vi "Acq&Buf-module5761.vi"(0 "DMATtoHOSTBlockNWords":u16, 1 "IntermediateFIFO":refnum<k21>="FIFO0", 2 "BUFFERS Info":T2={"CH0BUFFER"="CH0BUFFER", "CH1BUFFER"="CH1BUFFER", "CH2BUFFER"="CH2BUFFER", "CH3BUFFER"="CH3BUFFER", "CH0DMANumber "=0, "CH1DMANumber"=0, "CH2DMANumber"=0, "CH3DMANumber"=0}, 3 "DMA number":i32, 5 "SamplingRateN(DecimationFactor)":u16, 7 "NumberOfBuffers":T1, 9 "GroupEnableN":bool, 11 "DebugActivation":bool, 12 "Selected Channels":T4[](array[typedef])=[enum."Empty", enum."Empty", enum."Empty", enum."Empty"], 13 "NumChannels":T3) -> ()   [LabVIEW 2013, in "IRIO.lvlib"]
uses:
  IRIO.lvlib
  common/GlobalReg.vi
  <vilib>/eio/EIONode/EIONode.xnode
  <vilib>/rvi/eio/common/nirviEmuTemplateMethod_errors.vi
  <vilib>/rvi/DataTransferAndStorage/Container/XNode/niFpgaContainer.xnode
  <vilib>/rvi/FIFO/Fifo_Resource/niFpgaFifoEmulationRefIn.vi
  <vilib>/rvi/LocalResourceManager/LocalResourceManager.xnode
  <vilib>/rvi/DataTransferAndStorage/Container/Common/niFpgaContainerGetUniqueNameForEmu.vi
  <vilib>/rvi/DataTransferAndStorage/Container/Common/niFpgaContainerSetEmuInfo.vi
  <vilib>/rvi/eio/common/nirviEmuReportErrorAndStop.vi
  <vilib>/rvi/DataTransferAndStorage/Register/Emulation/niFpgaRegisterEmulationRefIn.vi
  ctl/SelectedChannels.ctl
  ctl/DMAConfigParams.ctl
  ctl/NumberOfBuffers.ctl
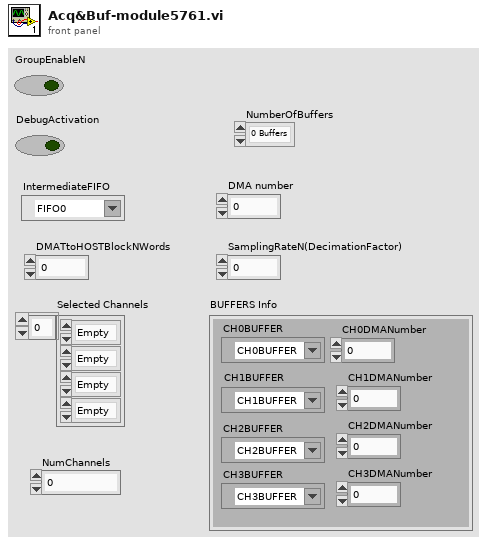
[diagram p1: front panel]
types:
  T1 = typedef "IRIO.lvlib/NumberOfBuffers.ctl" = enum16{"0 Buffers", "1 Buffers", "2 Buffers", "3 Buffers", "4 Buffers", "5 Buffers", "6 Buffers", "7 Buffers", "8 Buffers", "9 Buffers", "10 Buffers", "11 Buffers", "12 Buffers"}
  T2 = cluster{"CH0BUFFER":refnum<k21>, "CH1BUFFER":refnum<k21>, "CH2BUFFER":refnum<k21>, "CH3BUFFER":refnum<k21>, "CH0DMANumber ":i32, "CH1DMANumber":i32, "CH2DMANumber":i32, "CH3DMANumber":i32}
  T3 = typedef "IRIO.lvlib/DMAConfigParams.ctl" = u16
  T4 = typedef "IRIO.lvlib/SelectedChannels.ctl" = enum16{"Empty", "AI0", "AI1", "AI2", "AI3", "SignalGenerator0", "SignalGenerator1", "DDCA_PORT0", "DDCA_PORT1", "DDCA_PORT2", "DDCB_PORT0", "DDCB_PORT1", "DDCB_PORT2"}
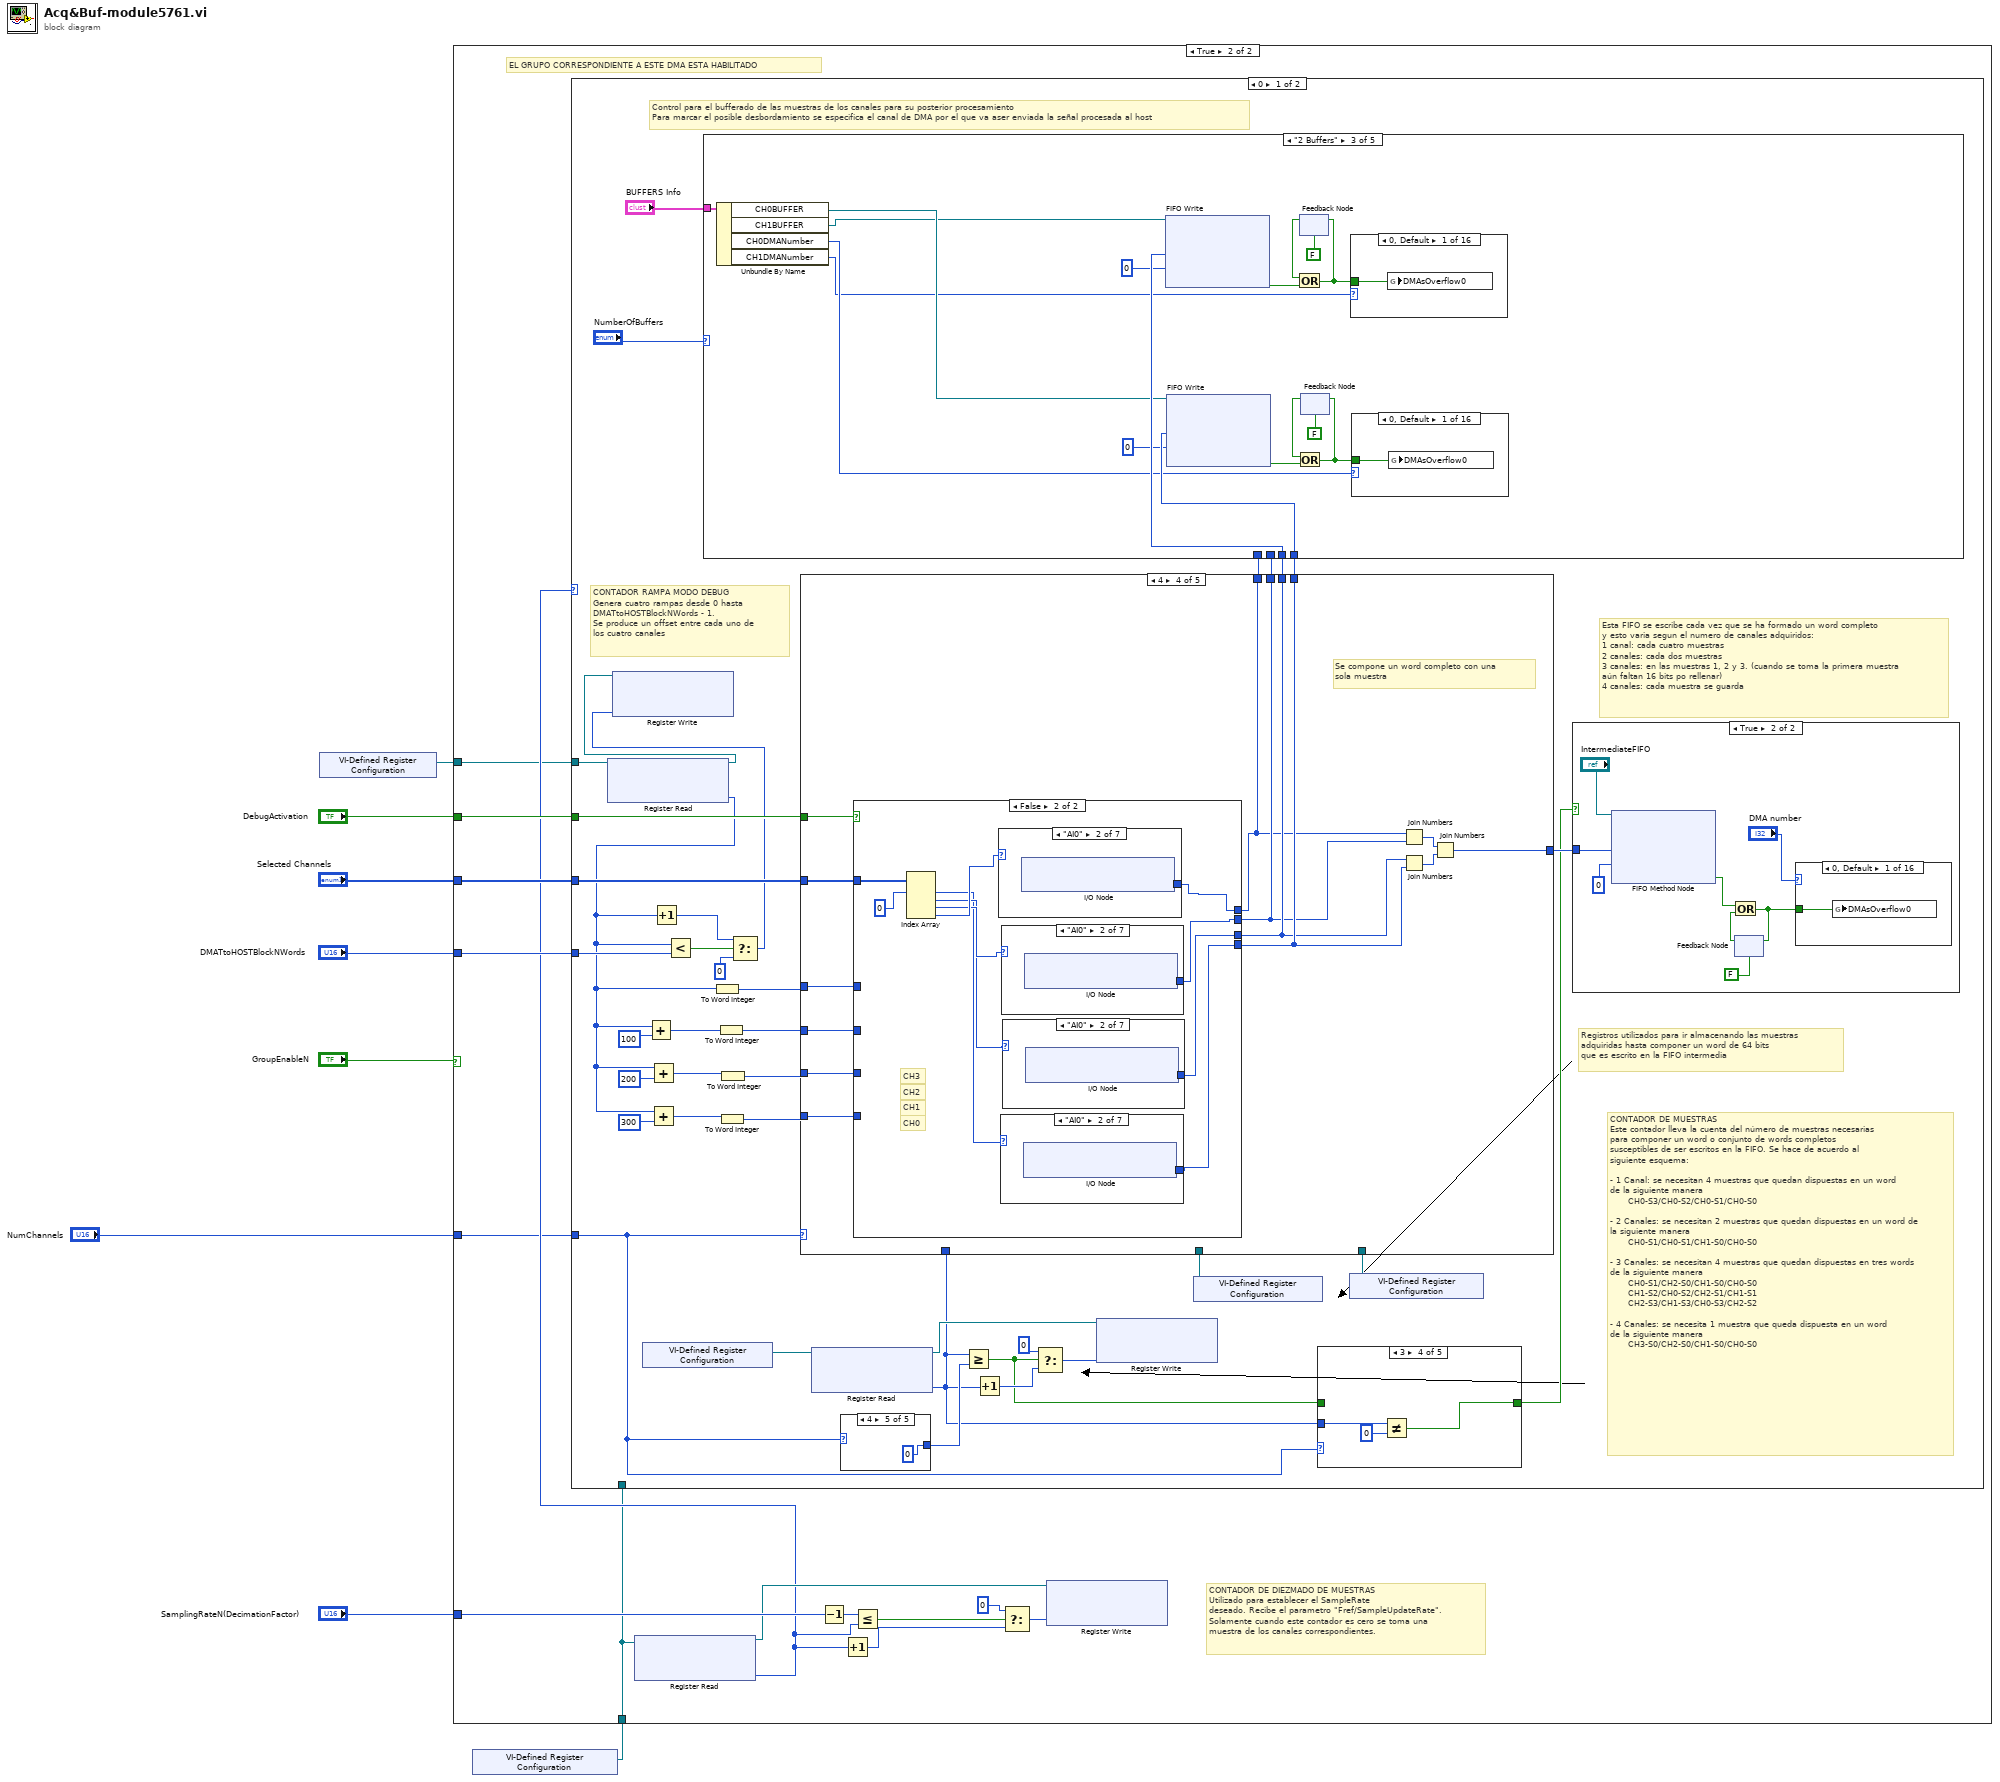
[diagram p0: block diagram]
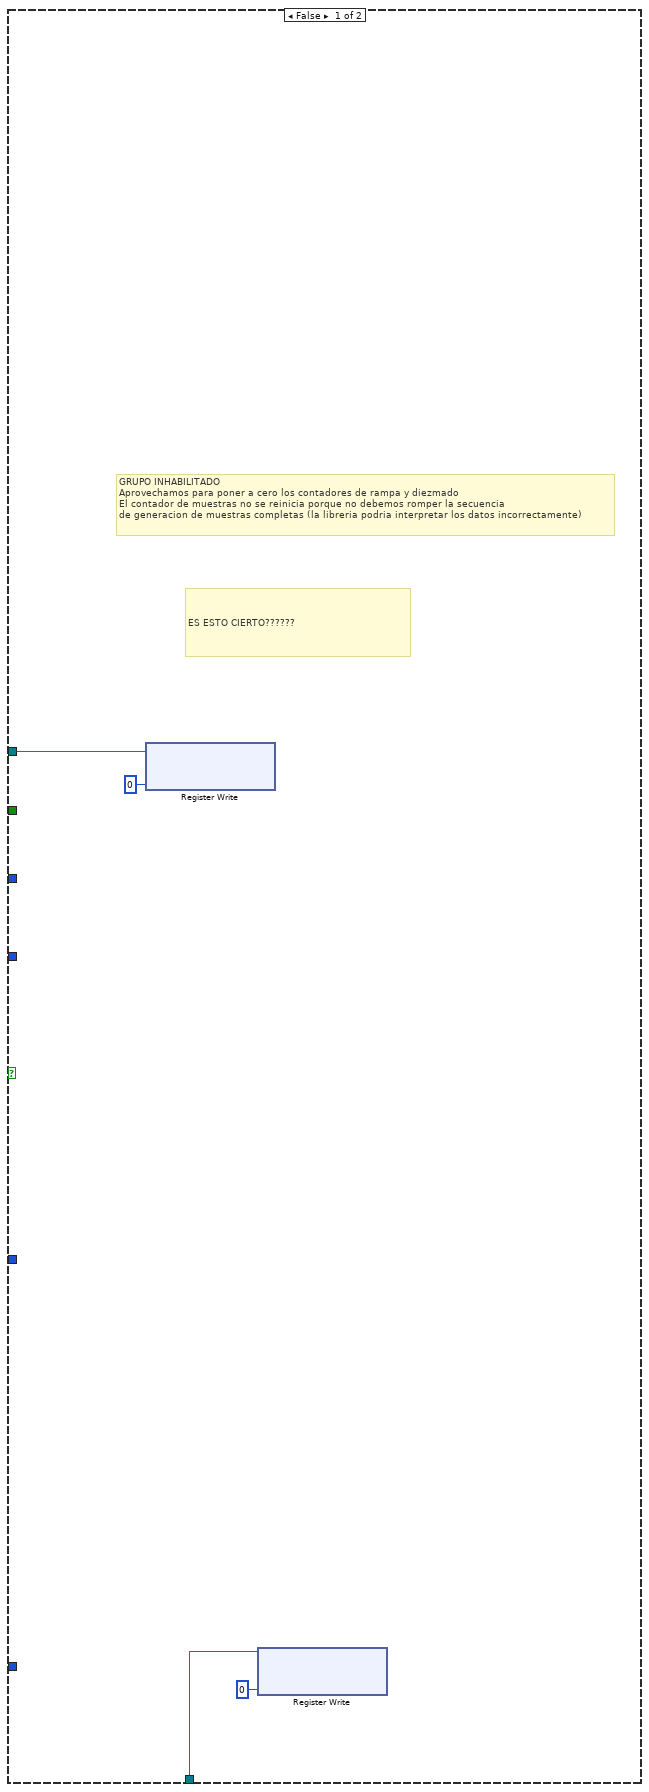
[diagram p2: hidden frame]
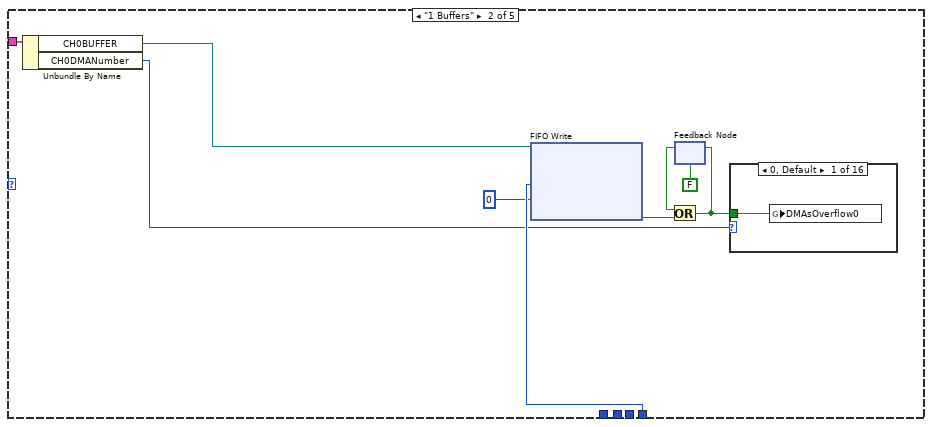
[diagram p4: hidden frame]
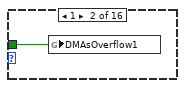
[diagram p5: hidden frame]
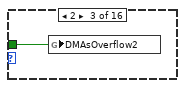
[diagram p6: hidden frame]
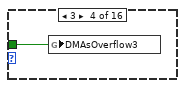
[diagram p7: hidden frame]
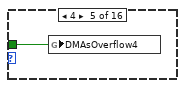
[diagram p8: hidden frame]
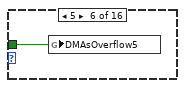
[diagram p9: hidden frame]
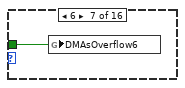
[diagram p10: hidden frame]
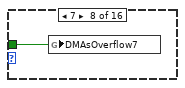
[diagram p11: hidden frame]
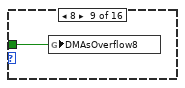
[diagram p12: hidden frame]
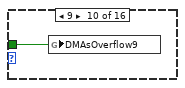
[diagram p13: hidden frame]
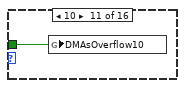
[diagram p14: hidden frame]
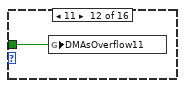
[diagram p15: hidden frame]
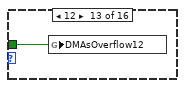
[diagram p16: hidden frame]
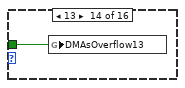
[diagram p17: hidden frame]
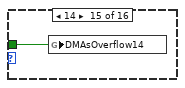
[diagram p18: hidden frame]
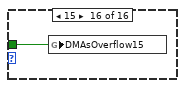
[diagram p19: hidden frame]
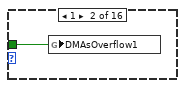
[diagram p20: hidden frame]
diagram:
  n1 = xnode ("VI-Defined Register Configuration")() -> ("Register Out"=w2:refnum<k21>)
  n2 = xnode ("VI-Defined Register Configuration")() -> ("Register Out"=w3:refnum<k21>)
  n3 = case shown="True" "GroupEnableN" {
    tunnel: "DebugActivation" -> [_ w26]
    tunnel: "DMATtoHOSTBlockNWords" -> [_ w25]
    tunnel: "NumChannels" -> [_ w13]
    tunnel: "Selected Channels" -> [_ w24]
    tunnel: "SamplingRateN(DecimationFactor)" -> [_ w19]
    tunnel: w3 -> [w12 w15]
    tunnel: w2 -> [w10 w14]
    frame False {
      # "ES ESTO CIERTO??????"
      # "GRUPO INHABILITADO\nAprovechamos para poner a cero los contadores de rampa y diezmado\nEl contador de muestras no se reinicia porque no debemos romper la secuencia\nde generacion de muestras completas (la libreria podria interpretar los datos incorrectamente)"
      n4 = xnode ("Register Write")("Data"=u16 0, "Register In"=w10) -> ()  [unwired: 1 out]
      n5 = xnode ("Register Write")("Data"=u16 0, "Register In"=w12) -> ()  [unwired: 1 out]
    }
    frame True {
      # "EL GRUPO CORRESPONDIENTE A ESTE DMA ESTA HABILITADO"
      # "CONTADOR DE DIEZMADO DE MUESTRAS\nUtilizado para establecer el SampleRate \ndeseado. Recibe el parametro \"Fref/SampleUpdateRate\".\nSolamente cuando este contador es cero se toma una\nmuestra de los canales correspondientes."
      n6 = xnode ("Register Read")("Register In"=w15) -> ("Register Out"=w18:refnum<k21>, "Data"=w16:u16)
      n7 = case shown="0" w16 {
        tunnel: w26 -> [w65 _]
        tunnel: w25 -> [w60 _]
        tunnel: w13 -> [w52 _]
        tunnel: w24 -> [w63 _]
        tunnel: w15 -> [_ _]
        tunnel: w14 -> [w45 _]
        frame 0 {
          # "Control para el bufferado de las muestras de los canales para su posterior procesamiento\nPara marcar el posible desbordamiento se especifica el canal de DMA por el que va aser enviada la señal procesada al host"
          # "Esta FIFO se escribe cada vez que se ha formado un word completo\ny esto varia segun el numero de canales adquiridos: \n1 canal: cada cuatro muestras\n2 canales: cada dos muestras\n3 canales: en las muestras 1, 2 y 3. (cuando se toma la primera muestra\naún faltan 16 bits po rellenar)\n4 canales: cada muestra se guarda"
          # "CONTADOR DE MUESTRAS\nEste contador lleva la cuenta del número de muestras necesarias\npara componer un word o conjunto de words completos\nsusceptibles de ser escritos en la FIFO. Se hace de acuerdo al\nsiguiente esquema:\n\n- 1 Canal: se necesitan 4 muestras que quedan dispuestas en un word \nde la siguiente manera\n      CH0-S3/CH0-S2/CH0-S1/CH0-S0\n\n- 2 Canales: se necesitan 2 muestras que quedan dispuestas en un word de la siguiente manera\n      CH0-S1/CH0-S1/CH1-S0/CH0-S0\n\n- 3 Canales: se necesitan 4 muestras que quedan dispuestas en tres words de la siguiente manera\n      CH0-S1/CH2-S0/CH1-S0/CH0-S0\n      CH1-S2/CH0-S2/CH2-S1/CH1-S1\n      CH2-S3/CH1-S3/CH0-S3/CH2-S2\n\n- 4 Canales: se necesita 1 muestra que queda dispuesta en un word \nde la siguiente manera\n      CH3-S0/CH2-S0/CH1-S0/CH0-S0"
          # "Registros utilizados para ir almacenando las muestras\nadquiridas hasta componer un word de 64 bits\nque es escrito en la FIFO intermedia"
          # "CONTADOR RAMPA MODO DEBUG\nGenera cuatro rampas desde 0 hasta \nDMATtoHOSTBlockNWords - 1.\nSe produce un offset entre cada uno de \nlos cuatro canales"
          n8 = xnode ("Register Read")("Register In"=w45) -> ("Data"=w33:u16, "Register Out"=w44:refnum<k21>)
          n9 = xnode ("VI-Defined Register Configuration")() -> ("Register Out"=w48:refnum<k21>)
          n10 = Add(x=w33, y=u16 100) -> (x+y=w40:u16)
          n11 = Add(x=w33, y=u16 200) -> (x+y=w38:u16)
          n12 = Add(x=w33, y=u16 300) -> (x+y=w36:u16)
          n13 = Increment(x=w33) -> (x+1=w62:u16)
          n14 = Less?(x=w33, y=w60) -> (x < y?=w61:bool)
          n15 = To Word Integer(number=w33) -> (16bit integer=w41:i16)
          n16 = To Word Integer(number=w40) -> (16bit integer=w39:i16)
          n17 = To Word Integer(number=w36) -> (16bit integer=w35:i16)
          n18 = To Word Integer(number=w38) -> (16bit integer=w37:i16)
          n19 = Select(t=w62, s=w61, f=u16 0) -> (s? t:f=w43:u16)
          n20 = xnode ("Register Write")("Data"=w43, "Register In"=w44) -> ()  [unwired: 1 out]
          n21 = xnode ("Register Read")("Register In"=w48) -> ("Register Out"=w53:refnum<k21>, "Data"=w49:u8)
          n22 = case shown="4" w52 {
            tunnel: [u8 0 u8 3 u8 1 u8 3 u8 0] -> w54
            frame 0, Default {
            }
            frame 1 {
            }
            frame 2 {
            }
            frame 3 {
            }
            frame 4 {
            }
          }
          n23 = Greater Or Equal?(x=w49, y=w54) -> (x >= y?=w51:bool)
          n24 = Increment(x=w49) -> (x+1=w57:u8)
          n25 = Select(t=u8 0 ("f"), s=w51, f=w57) -> (s? t:f=w55:u8)
          n26 = xnode ("Register Write")("Data"=w55, "Register In"=w53) -> ()  [unwired: 1 out]
          n27 = xnode ("VI-Defined Register Configuration")() -> ("Register Out"=w47:refnum<k21>)
          n28 = case shown="3" w52 {
            tunnel: w51 -> [_ w311 w312 _ w316]
            tunnel: [FALSE w311 w312 w313 w316] -> w50
            tunnel: w49 -> [_ _ _ w315 _]
            frame 0, Default {
            }
            frame 1 {
            }
            frame 2 {
            }
            frame 3 {
              n29 = Not Equal?(x=w315, y=u8 0) -> (x != y?=w313:bool)
            }
            frame 4 {
            }
          }
          n30 = xnode ("VI-Defined Register Configuration")() -> ("Register Out"=w46:refnum<k21>)
          n31 = case shown="4" w52 {
            tunnel: w65 -> [w354 w407 w459 w559 _]
            tunnel: w41 -> [w351 w404 w456 w558 _]
            tunnel: [w352 w405 w457 w554 u64 0] -> w64
            tunnel: w63 -> [w353 w406 w458 w557 _]
            tunnel: w39 -> [w350 w403 w455 w553 _]
            tunnel: w37 -> [_ _ w454 w552 _]
            tunnel: w35 -> [_ _ _ w551 _]
            tunnel: w49 -> [w349 w402 w453 _ _]
            tunnel: w47 -> [_ _ w452 _ _]
            tunnel: w46 -> [w348 w401 w451 _ _]
            tunnel: [w347 w400 w450 w550 w610] -> w32
            tunnel: [w346 w399 w449 w549 w610] -> w31
            tunnel: [w346 w398 w448 w548 w610] -> w30
            tunnel: [w346 w398 i16 0 ("IO Module\\AI 0") w547 w610] -> w29
            frame 1 {
              w346 = i16 0 ("IO Module\\AI 0")
              # "Cada muestra se va guardando en un registro intermedio\nhasta componer los 64 bits"
              n32 = case shown="False" w354 {
                tunnel: w353 -> [w357 _]
                tunnel: [w355 w368] -> w347
                tunnel: w351 -> [_ w368]
                tunnel: w350 -> [_ _]
                frame False {
                  n33 = Index Array(array=w357, index=0) -> (element=w356:T4)
                  n34 = case shown="\"AI0\"" w356 {
                    tunnel: [i16 0 ("IO Module\\AI 0") w360 w361 w362 w363 w365 w367] -> w355
                    frame "Empty", Default {
                    }
                    frame "AI0" {
                      n35 = xnode "I/O Node"() -> ("IO Module\\AI 0 Data N"=w360)  [unwired: 1 in, 1 out]
                    }
                    frame "AI1" {
                      n36 = xnode "I/O Node"() -> ("IO Module\\AI 1 Data N"=w361)  [unwired: 1 in, 1 out]
                    }
                    frame "AI2" {
                      n37 = xnode "I/O Node"() -> ("IO Module\\AI 2 Data N"=w362)  [unwired: 1 in, 1 out]
                    }
                    frame "AI3" {
                      n38 = xnode "I/O Node"() -> ("IO Module\\AI 3 Data N"=w363)  [unwired: 1 in, 1 out]
                    }
                    frame "SignalGenerator0" {
                      n39 = global read "GlobalReg.vi" "SimulatedAO0"() -> (w364:i32)
                      n40 = To Word Integer(number=w364) -> (16bit integer=w365:i16)
                    }
                    frame "SignalGenerator1" {
                      n41 = global read "GlobalReg.vi" "SimulatedAO1"() -> (w366:i32)
                      n42 = To Word Integer(number=w366) -> (16bit integer=w367:i16)
                    }
                  }
                }
                frame True {
                }
              }
              n43 = case shown="0, Default" w349 {
                tunnel: w347 -> [w371 w380 w387 w397]
                tunnel: [w370 w378 w385 w394] -> w352
                tunnel: w348 -> [w369 w377 w384 w392]
                frame 1 {
                  n44 = xnode ("Register Read")("Register In"=w369) -> ("Data"=w376:u64)  [unwired: 1 out]
                  n45 = Split Number(x=w376) -> (lo(x)=w375:u32)  [unwired: 1 out]
                  n46 = Split Number(x=w375) -> (lo(x)=w372:u16)  [unwired: 1 out]
                  n47 = Join Numbers(hi=w371, lo=w372) -> ((hi.lo)=w374:u32)
                  n48 = Join Numbers(hi=u32 0, lo=w374) -> ((hi.lo)=w370:u64)
                  n49 = xnode ("Register Write")("Data"=w370, "Register In"=w369) -> ()  [unwired: 1 out]
                }
                frame 2 {
                  n50 = xnode ("Register Read")("Register In"=w377) -> ("Data"=w383:u64)  [unwired: 1 out]
                  n51 = Split Number(x=w383) -> (lo(x)=w382:u32)  [unwired: 1 out]
                  n52 = Join Numbers(hi=u16 0, lo=w380) -> ((hi.lo)=w381:u32)
                  n53 = Join Numbers(hi=w381, lo=w382) -> ((hi.lo)=w378:u64)
                  n54 = xnode ("Register Write")("Data"=w378, "Register In"=w377) -> ()  [unwired: 1 out]
                }
                frame 3 {
                  n55 = xnode ("Register Read")("Register In"=w384) -> ("Data"=w391:u64)  [unwired: 1 out]
                  n56 = Split Number(x=w391) -> (hi(x)=w388:u32, lo(x)=w390:u32)
                  n57 = Split Number(x=w388) -> (lo(x)=w386:u16)  [unwired: 1 out]
                  n58 = Join Numbers(hi=w387, lo=w386) -> ((hi.lo)=w389:u32)
                  n59 = Join Numbers(hi=w389, lo=w390) -> ((hi.lo)=w385:u64)
                }
                frame 0, Default {
                  n60 = Join Numbers(hi=u16 0, lo=w397) -> ((hi.lo)=w396:u32)
                  n61 = Join Numbers(hi=u32 0, lo=w396) -> ((hi.lo)=w394:u64)
                  n62 = xnode ("Register Write")("Data"=w394, "Register In"=w392) -> ()  [unwired: 1 out]
                }
              }
            }
            frame 2 {
              w398 = i16 0 ("IO Module\\AI 0")
              # "Cada muestra de dos canales se van guardando en un registro\nintermedio hasta componer los 64 bits"
              n63 = case shown="False" w407 {
                tunnel: w406 -> [w412 _]
                tunnel: [w409 w433] -> w400
                tunnel: [w408 w432] -> w399
                tunnel: w404 -> [_ w433]
                tunnel: w403 -> [_ w432]
                frame False {
                  n64 = Index Array(array=w412, index #1=0 ("index")) -> (element #1=w411:T4, element #2=w410:T4)  [unwired: 1 in]
                  n65 = case shown="\"AI0\"" w411 {
                    tunnel: [i16 0 ("IO Module\\AI 0") w424 w425 w426 w427 w429 w431] -> w409
                    frame "Empty", Default {
                    }
                    frame "AI0" {
                      n66 = xnode "I/O Node"() -> ("IO Module\\AI 0 Data N"=w424)  [unwired: 1 in, 1 out]
                    }
                    frame "AI1" {
                      n67 = xnode "I/O Node"() -> ("IO Module\\AI 1 Data N"=w425)  [unwired: 1 in, 1 out]
                    }
                    frame "AI2" {
                      n68 = xnode "I/O Node"() -> ("IO Module\\AI 2 Data N"=w426)  [unwired: 1 in, 1 out]
                    }
                    frame "AI3" {
                      n69 = xnode "I/O Node"() -> ("IO Module\\AI 3 Data N"=w427)  [unwired: 1 in, 1 out]
                    }
                    frame "SignalGenerator0" {
                      n70 = global read "GlobalReg.vi" "SimulatedAO0"() -> (w428:i32)
                      n71 = To Word Integer(number=w428) -> (16bit integer=w429:i16)
                    }
                    frame "SignalGenerator1" {
                      n72 = global read "GlobalReg.vi" "SimulatedAO1"() -> (w430:i32)
                      n73 = To Word Integer(number=w430) -> (16bit integer=w431:i16)
                    }
                  }
                  n74 = case shown="\"AI0\"" w410 {
                    tunnel: [i16 0 ("IO Module\\AI 0") w415 w416 w417 w418 w420 w422] -> w408
                    frame "Empty", Default {
                    }
                    frame "AI0" {
                      n75 = xnode "I/O Node"() -> ("IO Module\\AI 0 Data N"=w415)  [unwired: 1 in, 1 out]
                    }
                    frame "AI1" {
                      n76 = xnode "I/O Node"() -> ("IO Module\\AI 1 Data N"=w416)  [unwired: 1 in, 1 out]
                    }
                    frame "AI2" {
                      n77 = xnode "I/O Node"() -> ("IO Module\\AI 2 Data N"=w417)  [unwired: 1 in, 1 out]
                    }
                    frame "AI3" {
                      n78 = xnode "I/O Node"() -> ("IO Module\\AI 3 Data N"=w418)  [unwired: 1 in, 1 out]
                    }
                    frame "SignalGenerator0" {
                      n79 = global read "GlobalReg.vi" "SimulatedAO0"() -> (w419:i32)
                      n80 = To Word Integer(number=w419) -> (16bit integer=w420:i16)
                    }
                    frame "SignalGenerator1" {
                      n81 = global read "GlobalReg.vi" "SimulatedAO1"() -> (w421:i32)
                      n82 = To Word Integer(number=w421) -> (16bit integer=w422:i16)
                    }
                  }
                }
                frame True {
                }
              }
              n83 = case shown="0, Default" w402 {
                tunnel: w400 -> [w440 w446]
                tunnel: w399 -> [w439 w445]
                tunnel: [w437 w442] -> w405
                tunnel: w401 -> [w434 w441]
                frame 1 {
                  n84 = xnode ("Register Read")("Register In"=w434) -> ("Data"=w438:u64)  [unwired: 1 out]
                  n85 = Join Numbers(hi=w439, lo=w440) -> ((hi.lo)=w435:u32)
                  n86 = Split Number(x=w438) -> (lo(x)=w436:u32)  [unwired: 1 out]
                  n87 = Join Numbers(hi=w435, lo=w436) -> ((hi.lo)=w437:u64)
                }
                frame 0, Default {
                  n88 = Join Numbers(hi=w445, lo=w446) -> ((hi.lo)=w444:u32)
                  n89 = Join Numbers(hi=u32 0, lo=w444) -> ((hi.lo)=w442:u64)
                  n90 = xnode ("Register Write")("Data"=w442, "Register In"=w441) -> ()  [unwired: 1 out]
                }
              }
            }
            frame 3 {
              # "Se necesitan dos registros porque las muestras de los tres canales\nen ocasiones quedan distribuidas entre dos word consecutivas. Cada\nuno de los tres words que se van generando se van escribiendo\nen la FIFO en el ciclo en el que se termina de componer"
              n91 = case shown="False" w459 {
                tunnel: w458 -> [w466 _]
                tunnel: [w465 w497] -> w450
                tunnel: [w464 w496] -> w449
                tunnel: w456 -> [_ w497]
                tunnel: w455 -> [_ w496]
                tunnel: [w463 w495] -> w448
                tunnel: w454 -> [_ w495]
                frame False {
                  n92 = Index Array(array=w466, index #1=0 ("index")) -> (element #1=w462:T4, element #2=w460:T4, element #3=w461:T4)  [unwired: 2 in]
                  n93 = case shown="\"AI0\"" w461 {
                    tunnel: [i16 0 ("IO Module\\AI 0") w469 w470 w471 w472 w474 w476] -> w463
                    frame "Empty", Default {
                    }
                    frame "AI0" {
                      n94 = xnode "I/O Node"() -> ("IO Module\\AI 0 Data N"=w469)  [unwired: 1 in, 1 out]
                    }
                    frame "AI1" {
                      n95 = xnode "I/O Node"() -> ("IO Module\\AI 1 Data N"=w470)  [unwired: 1 in, 1 out]
                    }
                    frame "AI2" {
                      n96 = xnode "I/O Node"() -> ("IO Module\\AI 2 Data N"=w471)  [unwired: 1 in, 1 out]
                    }
                    frame "AI3" {
                      n97 = xnode "I/O Node"() -> ("IO Module\\AI 3 Data N"=w472)  [unwired: 1 in, 1 out]
                    }
                    frame "SignalGenerator0" {
                      n98 = global read "GlobalReg.vi" "SimulatedAO0"() -> (w473:i32)
                      n99 = To Word Integer(number=w473) -> (16bit integer=w474:i16)
                    }
                    frame "SignalGenerator1" {
                      n100 = global read "GlobalReg.vi" "SimulatedAO1"() -> (w475:i32)
                      n101 = To Word Integer(number=w475) -> (16bit integer=w476:i16)
                    }
                  }
                  n102 = case shown="\"AI0\"" w462 {
                    tunnel: [i16 0 ("IO Module\\AI 0") w487 w488 w489 w490 w492 w494] -> w465
                    frame "Empty", Default {
                    }
                    frame "AI0" {
                      n103 = xnode "I/O Node"() -> ("IO Module\\AI 0 Data N"=w487)  [unwired: 1 in, 1 out]
                    }
                    frame "AI1" {
                      n104 = xnode "I/O Node"() -> ("IO Module\\AI 1 Data N"=w488)  [unwired: 1 in, 1 out]
                    }
                    frame "AI2" {
                      n105 = xnode "I/O Node"() -> ("IO Module\\AI 2 Data N"=w489)  [unwired: 1 in, 1 out]
                    }
                    frame "AI3" {
                      n106 = xnode "I/O Node"() -> ("IO Module\\AI 3 Data N"=w490)  [unwired: 1 in, 1 out]
                    }
                    frame "SignalGenerator0" {
                      n107 = global read "GlobalReg.vi" "SimulatedAO0"() -> (w491:i32)
                      n108 = To Word Integer(number=w491) -> (16bit integer=w492:i16)
                    }
                    frame "SignalGenerator1" {
                      n109 = global read "GlobalReg.vi" "SimulatedAO1"() -> (w493:i32)
                      n110 = To Word Integer(number=w493) -> (16bit integer=w494:i16)
                    }
                  }
                  n111 = case shown="\"AI0\"" w460 {
                    tunnel: [i16 0 ("IO Module\\AI 0") w478 w479 w480 w481 w483 w485] -> w464
                    frame "Empty", Default {
                    }
                    frame "AI0" {
                      n112 = xnode "I/O Node"() -> ("IO Module\\AI 0 Data N"=w478)  [unwired: 1 in, 1 out]
                    }
                    frame "AI1" {
                      n113 = xnode "I/O Node"() -> ("IO Module\\AI 1 Data N"=w479)  [unwired: 1 in, 1 out]
                    }
                    frame "AI2" {
                      n114 = xnode "I/O Node"() -> ("IO Module\\AI 2 Data N"=w480)  [unwired: 1 in, 1 out]
                    }
                    frame "AI3" {
                      n115 = xnode "I/O Node"() -> ("IO Module\\AI 3 Data N"=w481)  [unwired: 1 in, 1 out]
                    }
                    frame "SignalGenerator0" {
                      n116 = global read "GlobalReg.vi" "SimulatedAO0"() -> (w482:i32)
                      n117 = To Word Integer(number=w482) -> (16bit integer=w483:i16)
                    }
                    frame "SignalGenerator1" {
                      n118 = global read "GlobalReg.vi" "SimulatedAO1"() -> (w484:i32)
                      n119 = To Word Integer(number=w484) -> (16bit integer=w485:i16)
                    }
                  }
                }
                frame True {
                }
              }
              n120 = case shown="0, Default" w453 {
                tunnel: w450 -> [w507 w515 w528 w543]
                tunnel: w449 -> [w506 w510 w527 w538]
                tunnel: [w505 w521 w534 w546] -> w457
                tunnel: w448 -> [w502 w509 w526 w537]
                tunnel: w452 -> [w500 w514 w529 w542]
                tunnel: w451 -> [w498 w508 w523 w535]
                frame 0, Default {
                  # "No se lleva\nnada a la memoria\nde momento"
                  n121 = Join Numbers(hi=u16 0, lo=w502) -> ((hi.lo)=w503:u32)
                  n122 = Join Numbers(hi=w506, lo=w507) -> ((hi.lo)=w504:u32)
                  n123 = xnode ("Register Write")("Data"=u64 0, "Register In"=w500) -> ()  [unwired: 1 out]
                  n124 = Join Numbers(hi=w503, lo=w504) -> ((hi.lo)=w505:u64)
                  n125 = xnode ("Register Write")("Data"=w505, "Register In"=w498) -> ()  [unwired: 1 out]
                }
                frame 1 {
                  # "Listo registro 1"
                  n126 = Join Numbers(hi=w509, lo=w510) -> ((hi.lo)=w512:u32)
                  n127 = xnode ("Register Read")("Register In"=w508) -> ("Data"=w519:u64)  [unwired: 1 out]
                  n128 = Join Numbers(hi=u32 0, lo=w512) -> ((hi.lo)=w513:u64)
                  n129 = xnode ("Register Write")("Data"=w513, "Register In"=w514) -> ()  [unwired: 1 out]
                  n130 = Split Number(x=w519) -> (hi(x)=w517:u32, lo(x)=w518:u32)
                  n131 = Split Number(x=w517) -> (lo(x)=w516:u16)  [unwired: 1 out]
                  n132 = Join Numbers(hi=w515, lo=w516) -> ((hi.lo)=w520:u32)
                  n133 = Join Numbers(hi=w520, lo=w518) -> ((hi.lo)=w521:u64)
                }
                frame 2 {
                  # "Listo registro 2"
                  n134 = Join Numbers(hi=u16 0, lo=w526) -> ((hi.lo)=w530:u32)
                  n135 = xnode ("Register Read")("Register In"=w529) -> ("Data"=w532:u64)  [unwired: 1 out]
                  n136 = Join Numbers(hi=u32 0, lo=w530) -> ((hi.lo)=w524:u64)
                  n137 = xnode ("Register Write")("Data"=w524, "Register In"=w523) -> ()  [unwired: 1 out]
                  n138 = Split Number(x=w532) -> (lo(x)=w531:u32)  [unwired: 1 out]
                  n139 = Join Numbers(hi=w527, lo=w528) -> ((hi.lo)=w533:u32)
                  n140 = Join Numbers(hi=w533, lo=w531) -> ((hi.lo)=w534:u64)
                }
                frame 3 {
                  # "Listo registro 1"
                  n141 = xnode ("Register Read")("Register In"=w535) -> ("Data"=w545:u64)  [unwired: 1 out]
                  n142 = xnode ("Register Write")("Data"=u64 0 ("hi"), "Register In"=w542) -> ()  [unwired: 1 out]
                  n143 = Split Number(x=w545) -> (lo(x)=w540:u32)  [unwired: 1 out]
                  n144 = Split Number(x=w540) -> (lo(x)=w544:u16)  [unwired: 1 out]
                  n145 = Join Numbers(hi=w537, lo=w538) -> ((hi.lo)=w536:u32)
                  n146 = Join Numbers(hi=w543, lo=w544) -> ((hi.lo)=w539:u32)
                  n147 = Join Numbers(hi=w536, lo=w539) -> ((hi.lo)=w546:u64)
                }
              }
            }
            frame 4 {
              # "Se compone un word completo con una\nsola muestra"
              n148 = case shown="False" w559 {
                tunnel: w558 -> [w563 _]
                tunnel: w557 -> [_ w572]
                tunnel: [w560 w567] -> w547
                tunnel: [w561 w566] -> w548
                tunnel: [w562 w565] -> w549
                tunnel: [w563 w564] -> w550
                tunnel: w553 -> [w562 _]
                tunnel: w552 -> [w561 _]
                tunnel: w551 -> [w560 _]
                frame True {
                }
                frame False {
                  # "CH0"
                  # "CH1"
                  # "CH2"
                  # "CH3"
                  n149 = Index Array(array=w572, index #1=0 ("index")) -> (element #1=w568:T4, element #2=w569:T4, element #3=w570:T4, element #4=w571:T4)  [unwired: 3 in]
                  n150 = case shown="\"AI0\"" w571 {
                    tunnel: [i16 0 ("IO Module\\AI 0") w575 w576 w577 w578 w580 w582] -> w567
                    frame "Empty", Default {
                    }
                    frame "AI0" {
                      n151 = xnode "I/O Node"() -> ("IO Module\\AI 0 Data N"=w575)  [unwired: 1 in, 1 out]
                    }
                    frame "AI1" {
                      n152 = xnode "I/O Node"() -> ("IO Module\\AI 1 Data N"=w576)  [unwired: 1 in, 1 out]
                    }
                    frame "AI2" {
                      n153 = xnode "I/O Node"() -> ("IO Module\\AI 2 Data N"=w577)  [unwired: 1 in, 1 out]
                    }
                    frame "AI3" {
                      n154 = xnode "I/O Node"() -> ("IO Module\\AI 3 Data N"=w578)  [unwired: 1 in, 1 out]
                    }
                    frame "SignalGenerator0" {
                      n155 = global read "GlobalReg.vi" "SimulatedAO0"() -> (w579:i32)
                      n156 = To Word Integer(number=w579) -> (16bit integer=w580:i16)
                    }
                    frame "SignalGenerator1" {
                      n157 = global read "GlobalReg.vi" "SimulatedAO1"() -> (w581:i32)
                      n158 = To Word Integer(number=w581) -> (16bit integer=w582:i16)
                    }
                  }
                  n159 = case shown="\"AI0\"" w568 {
                    tunnel: [i16 0 ("IO Module\\AI 0") w602 w603 w604 w605 w607 w609] -> w564
                    frame "Empty", Default {
                    }
                    frame "AI0" {
                      n160 = xnode "I/O Node"() -> ("IO Module\\AI 0 Data N"=w602)  [unwired: 1 in, 1 out]
                    }
                    frame "AI1" {
                      n161 = xnode "I/O Node"() -> ("IO Module\\AI 1 Data N"=w603)  [unwired: 1 in, 1 out]
                    }
                    frame "AI2" {
                      n162 = xnode "I/O Node"() -> ("IO Module\\AI 2 Data N"=w604)  [unwired: 1 in, 1 out]
                    }
                    frame "AI3" {
                      n163 = xnode "I/O Node"() -> ("IO Module\\AI 3 Data N"=w605)  [unwired: 1 in, 1 out]
                    }
                    frame "SignalGenerator0" {
                      n164 = global read "GlobalReg.vi" "SimulatedAO0"() -> (w606:i32)
                      n165 = To Word Integer(number=w606) -> (16bit integer=w607:i16)
                    }
                    frame "SignalGenerator1" {
                      n166 = global read "GlobalReg.vi" "SimulatedAO1"() -> (w608:i32)
                      n167 = To Word Integer(number=w608) -> (16bit integer=w609:i16)
                    }
                  }
                  n168 = case shown="\"AI0\"" w570 {
                    tunnel: [i16 0 ("IO Module\\AI 0") w584 w585 w586 w587 w589 w591] -> w566
                    frame "Empty", Default {
                    }
                    frame "AI0" {
                      n169 = xnode "I/O Node"() -> ("IO Module\\AI 0 Data N"=w584)  [unwired: 1 in, 1 out]
                    }
                    frame "AI1" {
                      n170 = xnode "I/O Node"() -> ("IO Module\\AI 1 Data N"=w585)  [unwired: 1 in, 1 out]
                    }
                    frame "AI2" {
                      n171 = xnode "I/O Node"() -> ("IO Module\\AI 2 Data N"=w586)  [unwired: 1 in, 1 out]
                    }
                    frame "AI3" {
                      n172 = xnode "I/O Node"() -> ("IO Module\\AI 3 Data N"=w587)  [unwired: 1 in, 1 out]
                    }
                    frame "SignalGenerator0" {
                      n173 = global read "GlobalReg.vi" "SimulatedAO0"() -> (w588:i32)
                      n174 = To Word Integer(number=w588) -> (16bit integer=w589:i16)
                    }
                    frame "SignalGenerator1" {
                      n175 = global read "GlobalReg.vi" "SimulatedAO1"() -> (w590:i32)
                      n176 = To Word Integer(number=w590) -> (16bit integer=w591:i16)
                    }
                  }
                  n177 = case shown="\"AI0\"" w569 {
                    tunnel: [i16 0 ("IO Module\\AI 0") w593 w594 w595 w596 w598 w600] -> w565
                    frame "Empty", Default {
                    }
                    frame "AI0" {
                      n178 = xnode "I/O Node"() -> ("IO Module\\AI 0 Data N"=w593)  [unwired: 1 in, 1 out]
                    }
                    frame "AI1" {
                      n179 = xnode "I/O Node"() -> ("IO Module\\AI 1 Data N"=w594)  [unwired: 1 in, 1 out]
                    }
                    frame "AI2" {
                      n180 = xnode "I/O Node"() -> ("IO Module\\AI 2 Data N"=w595)  [unwired: 1 in, 1 out]
                    }
                    frame "AI3" {
                      n181 = xnode "I/O Node"() -> ("IO Module\\AI 3 Data N"=w596)  [unwired: 1 in, 1 out]
                    }
                    frame "SignalGenerator0" {
                      n182 = global read "GlobalReg.vi" "SimulatedAO0"() -> (w597:i32)
                      n183 = To Word Integer(number=w597) -> (16bit integer=w598:i16)
                    }
                    frame "SignalGenerator1" {
                      n184 = global read "GlobalReg.vi" "SimulatedAO1"() -> (w599:i32)
                      n185 = To Word Integer(number=w599) -> (16bit integer=w600:i16)
                    }
                  }
                }
              }
              n186 = Join Numbers(hi=w547, lo=w548) -> ((hi.lo)=w556:u32)
              n187 = Join Numbers(hi=w549, lo=w550) -> ((hi.lo)=w555:u32)
              n188 = Join Numbers(hi=w556, lo=w555) -> ((hi.lo)=w554:u64)
            }
            frame Default {
              w610 = i16 0 ("IO Module\\AI 0")
            }
          }
          n189 = case shown="\"2 Buffers\"" "NumberOfBuffers" {
            tunnel: w32 -> [_ w74 w107 w164 w245]
            tunnel: w31 -> [_ _ w106 w163 w244]
            tunnel: w30 -> [_ _ _ w162 w243]
            tunnel: w29 -> [_ _ _ _ w242]
            tunnel: "BUFFERS Info" -> [_ w73 w105 w161 w241]
            frame "0 Buffers", Default {
            }
            frame "1 Buffers" {
              n190 = Unbundle By Name(w73) -> ("CH0BUFFER"=w72:refnum<k21>, "CH0DMANumber"=w71:i32)
              n191 = xnode ("FIFO Write")("Element"=w74, "Timeout"=0, "FIFO In"=w72) -> ("Timed Out?"=w66:bool)  [unwired: 1 out]
              n192 = feedback #1(FALSE) -> (w68:bool)
              n193 = Or(x=w68, y=w66) -> (x .or. y?=w69:bool)
              n194 = feedback-in #1(w69) -> ()
              n195 = case shown="0, Default" w71 {
                tunnel: w69 -> [w75 w76 w77 w78 w79 w80 w81 w82 w83 w84 w85 w86 w87 w88 w89 w90]
                frame 0, Default {
                  n196 = global write "GlobalReg.vi" "DMAsOverflow0"(w75) -> ()
                }
                frame 1 {
                  n197 = global write "GlobalReg.vi" "DMAsOverflow1"(w76) -> ()
                }
                frame 2 {
                  n198 = global write "GlobalReg.vi" "DMAsOverflow2"(w77) -> ()
                }
                frame 3 {
                  n199 = global write "GlobalReg.vi" "DMAsOverflow3"(w78) -> ()
                }
                frame 4 {
                  n200 = global write "GlobalReg.vi" "DMAsOverflow4"(w79) -> ()
                }
                frame 5 {
                  n201 = global write "GlobalReg.vi" "DMAsOverflow5"(w80) -> ()
                }
                frame 6 {
                  n202 = global write "GlobalReg.vi" "DMAsOverflow6"(w81) -> ()
                }
                frame 7 {
                  n203 = global write "GlobalReg.vi" "DMAsOverflow7"(w82) -> ()
                }
                frame 8 {
                  n204 = global write "GlobalReg.vi" "DMAsOverflow8"(w83) -> ()
                }
                frame 9 {
                  n205 = global write "GlobalReg.vi" "DMAsOverflow9"(w84) -> ()
                }
                frame 10 {
                  n206 = global write "GlobalReg.vi" "DMAsOverflow10"(w85) -> ()
                }
                frame 11 {
                  n207 = global write "GlobalReg.vi" "DMAsOverflow11"(w86) -> ()
                }
                frame 12 {
                  n208 = global write "GlobalReg.vi" "DMAsOverflow12"(w87) -> ()
                }
                frame 13 {
                  n209 = global write "GlobalReg.vi" "DMAsOverflow13"(w88) -> ()
                }
                frame 14 {
                  n210 = global write "GlobalReg.vi" "DMAsOverflow14"(w89) -> ()
                }
                frame 15 {
                  n211 = global write "GlobalReg.vi" "DMAsOverflow15"(w90) -> ()
                }
              }
            }
            frame "2 Buffers" {
              n212 = Unbundle By Name(w105) -> ("CH0BUFFER"=w104:refnum<k21>, "CH1BUFFER"=w103:refnum<k21>, "CH0DMANumber"=w102:i32, "CH1DMANumber"=w101:i32)
              n213 = xnode ("FIFO Write")("Element"=w106, "Timeout"=0, "FIFO In"=w103) -> ("Timed Out?"=w96:bool)  [unwired: 1 out]
              n214 = xnode ("FIFO Write")("Element"=w107, "Timeout"=0, "FIFO In"=w104) -> ("Timed Out?"=w91:bool)  [unwired: 1 out]
              n215 = feedback #2(FALSE) -> (w98:bool)
              n216 = Or(x=w98, y=w96) -> (x .or. y?=w99:bool)
              n217 = feedback-in #2(w99) -> ()
              n218 = feedback #3(FALSE) -> (w93:bool)
              n219 = Or(x=w93, y=w91) -> (x .or. y?=w94:bool)
              n220 = feedback-in #3(w94) -> ()
              n221 = case shown="0, Default" w101 {
                tunnel: w99 -> [w124 w125 w126 w127 w128 w129 w130 w131 w132 w133 w134 w135 w136 w137 w138 w139]
                frame 0, Default {
                  n222 = global write "GlobalReg.vi" "DMAsOverflow0"(w124) -> ()
                }
                frame 1 {
                  n223 = global write "GlobalReg.vi" "DMAsOverflow1"(w125) -> ()
                }
                frame 2 {
                  n224 = global write "GlobalReg.vi" "DMAsOverflow2"(w126) -> ()
                }
                frame 3 {
                  n225 = global write "GlobalReg.vi" "DMAsOverflow3"(w127) -> ()
                }
                frame 4 {
                  n226 = global write "GlobalReg.vi" "DMAsOverflow4"(w128) -> ()
                }
                frame 5 {
                  n227 = global write "GlobalReg.vi" "DMAsOverflow5"(w129) -> ()
                }
                frame 6 {
                  n228 = global write "GlobalReg.vi" "DMAsOverflow6"(w130) -> ()
                }
                frame 7 {
                  n229 = global write "GlobalReg.vi" "DMAsOverflow7"(w131) -> ()
                }
                frame 8 {
                  n230 = global write "GlobalReg.vi" "DMAsOverflow8"(w132) -> ()
                }
                frame 9 {
                  n231 = global write "GlobalReg.vi" "DMAsOverflow9"(w133) -> ()
                }
                frame 10 {
                  n232 = global write "GlobalReg.vi" "DMAsOverflow10"(w134) -> ()
                }
                frame 11 {
                  n233 = global write "GlobalReg.vi" "DMAsOverflow11"(w135) -> ()
                }
                frame 12 {
                  n234 = global write "GlobalReg.vi" "DMAsOverflow12"(w136) -> ()
                }
                frame 13 {
                  n235 = global write "GlobalReg.vi" "DMAsOverflow13"(w137) -> ()
                }
                frame 14 {
                  n236 = global write "GlobalReg.vi" "DMAsOverflow14"(w138) -> ()
                }
                frame 15 {
                  n237 = global write "GlobalReg.vi" "DMAsOverflow15"(w139) -> ()
                }
              }
              n238 = case shown="0, Default" w102 {
                tunnel: w94 -> [w108 w109 w110 w111 w112 w113 w114 w115 w116 w117 w118 w119 w120 w121 w122 w123]
                frame 0, Default {
                  n239 = global write "GlobalReg.vi" "DMAsOverflow0"(w108) -> ()
                }
                frame 1 {
                  n240 = global write "GlobalReg.vi" "DMAsOverflow1"(w109) -> ()
                }
                frame 2 {
                  n241 = global write "GlobalReg.vi" "DMAsOverflow2"(w110) -> ()
                }
                frame 3 {
                  n242 = global write "GlobalReg.vi" "DMAsOverflow3"(w111) -> ()
                }
                frame 4 {
                  n243 = global write "GlobalReg.vi" "DMAsOverflow4"(w112) -> ()
                }
                frame 5 {
                  n244 = global write "GlobalReg.vi" "DMAsOverflow5"(w113) -> ()
                }
                frame 6 {
                  n245 = global write "GlobalReg.vi" "DMAsOverflow6"(w114) -> ()
                }
                frame 7 {
                  n246 = global write "GlobalReg.vi" "DMAsOverflow7"(w115) -> ()
                }
                frame 8 {
                  n247 = global write "GlobalReg.vi" "DMAsOverflow8"(w116) -> ()
                }
                frame 9 {
                  n248 = global write "GlobalReg.vi" "DMAsOverflow9"(w117) -> ()
                }
                frame 10 {
                  n249 = global write "GlobalReg.vi" "DMAsOverflow10"(w118) -> ()
                }
                frame 11 {
                  n250 = global write "GlobalReg.vi" "DMAsOverflow11"(w119) -> ()
                }
                frame 12 {
                  n251 = global write "GlobalReg.vi" "DMAsOverflow12"(w120) -> ()
                }
                frame 13 {
                  n252 = global write "GlobalReg.vi" "DMAsOverflow13"(w121) -> ()
                }
                frame 14 {
                  n253 = global write "GlobalReg.vi" "DMAsOverflow14"(w122) -> ()
                }
                frame 15 {
                  n254 = global write "GlobalReg.vi" "DMAsOverflow15"(w123) -> ()
                }
              }
            }
            frame "3 Buffers" {
              n255 = Unbundle By Name(w161) -> ("CH0BUFFER"=w159:refnum<k21>, "CH1BUFFER"=w158:refnum<k21>, "CH2BUFFER"=w160:refnum<k21>, "CH0DMANumber"=w157:i32, "CH1DMANumber"=w156:i32, "CH2DMANumber"=w155:i32)
              n256 = xnode ("FIFO Write")("Element"=w162, "Timeout"=0, "FIFO In"=w160) -> ("Timed Out?"=w150:bool)  [unwired: 1 out]
              n257 = feedback #4(FALSE) -> (w152:bool)
              n258 = Or(x=w152, y=w150) -> (x .or. y?=w153:bool)
              n259 = feedback-in #4(w153) -> ()
              n260 = case shown="0, Default" w155 {
                tunnel: w153 -> [w197 w198 w199 w200 w201 w202 w203 w204 w205 w206 w207 w208 w209 w210 w211 w212]
                frame 0, Default {
                  n261 = global write "GlobalReg.vi" "DMAsOverflow0"(w197) -> ()
                }
                frame 1 {
                  n262 = global write "GlobalReg.vi" "DMAsOverflow1"(w198) -> ()
                }
                frame 2 {
                  n263 = global write "GlobalReg.vi" "DMAsOverflow2"(w199) -> ()
                }
                frame 3 {
                  n264 = global write "GlobalReg.vi" "DMAsOverflow3"(w200) -> ()
                }
                frame 4 {
                  n265 = global write "GlobalReg.vi" "DMAsOverflow4"(w201) -> ()
                }
                frame 5 {
                  n266 = global write "GlobalReg.vi" "DMAsOverflow5"(w202) -> ()
                }
                frame 6 {
                  n267 = global write "GlobalReg.vi" "DMAsOverflow6"(w203) -> ()
                }
                frame 7 {
                  n268 = global write "GlobalReg.vi" "DMAsOverflow7"(w204) -> ()
                }
                frame 8 {
                  n269 = global write "GlobalReg.vi" "DMAsOverflow8"(w205) -> ()
                }
                frame 9 {
                  n270 = global write "GlobalReg.vi" "DMAsOverflow9"(w206) -> ()
                }
                frame 10 {
                  n271 = global write "GlobalReg.vi" "DMAsOverflow10"(w207) -> ()
                }
                frame 11 {
                  n272 = global write "GlobalReg.vi" "DMAsOverflow11"(w208) -> ()
                }
                frame 12 {
                  n273 = global write "GlobalReg.vi" "DMAsOverflow12"(w209) -> ()
                }
                frame 13 {
                  n274 = global write "GlobalReg.vi" "DMAsOverflow13"(w210) -> ()
                }
                frame 14 {
                  n275 = global write "GlobalReg.vi" "DMAsOverflow14"(w211) -> ()
                }
                frame 15 {
                  n276 = global write "GlobalReg.vi" "DMAsOverflow15"(w212) -> ()
                }
              }
              n277 = xnode ("FIFO Write")("Element"=w163, "Timeout"=0, "FIFO In"=w158) -> ("Timed Out?"=w145:bool)  [unwired: 1 out]
              n278 = xnode ("FIFO Write")("Element"=w164, "Timeout"=0, "FIFO In"=w159) -> ("Timed Out?"=w140:bool)  [unwired: 1 out]
              n279 = feedback #5(FALSE) -> (w147:bool)
              n280 = Or(x=w147, y=w145) -> (x .or. y?=w148:bool)
              n281 = feedback-in #5(w148) -> ()
              n282 = feedback #6(FALSE) -> (w142:bool)
              n283 = Or(x=w142, y=w140) -> (x .or. y?=w143:bool)
              n284 = feedback-in #6(w143) -> ()
              n285 = case shown="0, Default" w156 {
                tunnel: w148 -> [w181 w182 w183 w184 w185 w186 w187 w188 w189 w190 w191 w192 w193 w194 w195 w196]
                frame 0, Default {
                  n286 = global write "GlobalReg.vi" "DMAsOverflow0"(w181) -> ()
                }
                frame 1 {
                  n287 = global write "GlobalReg.vi" "DMAsOverflow1"(w182) -> ()
                }
                frame 2 {
                  n288 = global write "GlobalReg.vi" "DMAsOverflow2"(w183) -> ()
                }
                frame 3 {
                  n289 = global write "GlobalReg.vi" "DMAsOverflow3"(w184) -> ()
                }
                frame 4 {
                  n290 = global write "GlobalReg.vi" "DMAsOverflow4"(w185) -> ()
                }
                frame 5 {
                  n291 = global write "GlobalReg.vi" "DMAsOverflow5"(w186) -> ()
                }
                frame 6 {
                  n292 = global write "GlobalReg.vi" "DMAsOverflow6"(w187) -> ()
                }
                frame 7 {
                  n293 = global write "GlobalReg.vi" "DMAsOverflow7"(w188) -> ()
                }
                frame 8 {
                  n294 = global write "GlobalReg.vi" "DMAsOverflow8"(w189) -> ()
                }
                frame 9 {
                  n295 = global write "GlobalReg.vi" "DMAsOverflow9"(w190) -> ()
                }
                frame 10 {
                  n296 = global write "GlobalReg.vi" "DMAsOverflow10"(w191) -> ()
                }
                frame 11 {
                  n297 = global write "GlobalReg.vi" "DMAsOverflow11"(w192) -> ()
                }
                frame 12 {
                  n298 = global write "GlobalReg.vi" "DMAsOverflow12"(w193) -> ()
                }
                frame 13 {
                  n299 = global write "GlobalReg.vi" "DMAsOverflow13"(w194) -> ()
                }
                frame 14 {
                  n300 = global write "GlobalReg.vi" "DMAsOverflow14"(w195) -> ()
                }
                frame 15 {
                  n301 = global write "GlobalReg.vi" "DMAsOverflow15"(w196) -> ()
                }
              }
              n302 = case shown="0, Default" w157 {
                tunnel: w143 -> [w165 w166 w167 w168 w169 w170 w171 w172 w173 w174 w175 w176 w177 w178 w179 w180]
                frame 0, Default {
                  n303 = global write "GlobalReg.vi" "DMAsOverflow0"(w165) -> ()
                }
                frame 1 {
                  n304 = global write "GlobalReg.vi" "DMAsOverflow1"(w166) -> ()
                }
                frame 2 {
                  n305 = global write "GlobalReg.vi" "DMAsOverflow2"(w167) -> ()
                }
                frame 3 {
                  n306 = global write "GlobalReg.vi" "DMAsOverflow3"(w168) -> ()
                }
                frame 4 {
                  n307 = global write "GlobalReg.vi" "DMAsOverflow4"(w169) -> ()
                }
                frame 5 {
                  n308 = global write "GlobalReg.vi" "DMAsOverflow5"(w170) -> ()
                }
                frame 6 {
                  n309 = global write "GlobalReg.vi" "DMAsOverflow6"(w171) -> ()
                }
                frame 7 {
                  n310 = global write "GlobalReg.vi" "DMAsOverflow7"(w172) -> ()
                }
                frame 8 {
                  n311 = global write "GlobalReg.vi" "DMAsOverflow8"(w173) -> ()
                }
                frame 9 {
                  n312 = global write "GlobalReg.vi" "DMAsOverflow9"(w174) -> ()
                }
                frame 10 {
                  n313 = global write "GlobalReg.vi" "DMAsOverflow10"(w175) -> ()
                }
                frame 11 {
                  n314 = global write "GlobalReg.vi" "DMAsOverflow11"(w176) -> ()
                }
                frame 12 {
                  n315 = global write "GlobalReg.vi" "DMAsOverflow12"(w177) -> ()
                }
                frame 13 {
                  n316 = global write "GlobalReg.vi" "DMAsOverflow13"(w178) -> ()
                }
                frame 14 {
                  n317 = global write "GlobalReg.vi" "DMAsOverflow14"(w179) -> ()
                }
                frame 15 {
                  n318 = global write "GlobalReg.vi" "DMAsOverflow15"(w180) -> ()
                }
              }
            }
            frame "4 Buffers" {
              n319 = Unbundle By Name(w241) -> ("CH0BUFFER"=w236:refnum<k21>, "CH1BUFFER"=w235:refnum<k21>, "CH2BUFFER"=w239:refnum<k21>, "CH3BUFFER"=w240:refnum<k21>, "CH0DMANumber"=w234:i32, "CH1DMANumber"=w233:i32, "CH2DMANumber"=w237:i32, "CH3DMANumber"=w238:i32)
              n320 = xnode ("FIFO Write")("Element"=w242, "Timeout"=0, "FIFO In"=w240) -> ("Timed Out?"=w228:bool)  [unwired: 1 out]
              n321 = xnode ("FIFO Write")("Element"=w243, "Timeout"=0, "FIFO In"=w239) -> ("Timed Out?"=w223:bool)  [unwired: 1 out]
              n322 = feedback #7(FALSE) -> (w230:bool)
              n323 = Or(x=w230, y=w228) -> (x .or. y?=w231:bool)
              n324 = feedback-in #7(w231) -> ()
              n325 = feedback #8(FALSE) -> (w225:bool)
              n326 = Or(x=w225, y=w223) -> (x .or. y?=w226:bool)
              n327 = feedback-in #8(w226) -> ()
              n328 = case shown="0, Default" w238 {
                tunnel: w231 -> [w294 w295 w296 w297 w298 w299 w300 w301 w302 w303 w304 w305 w306 w307 w308 w309]
                frame 0, Default {
                  n329 = global write "GlobalReg.vi" "DMAsOverflow0"(w294) -> ()
                }
                frame 1 {
                  n330 = global write "GlobalReg.vi" "DMAsOverflow1"(w295) -> ()
                }
                frame 2 {
                  n331 = global write "GlobalReg.vi" "DMAsOverflow2"(w296) -> ()
                }
                frame 3 {
                  n332 = global write "GlobalReg.vi" "DMAsOverflow3"(w297) -> ()
                }
                frame 4 {
                  n333 = global write "GlobalReg.vi" "DMAsOverflow4"(w298) -> ()
                }
                frame 5 {
                  n334 = global write "GlobalReg.vi" "DMAsOverflow5"(w299) -> ()
                }
                frame 6 {
                  n335 = global write "GlobalReg.vi" "DMAsOverflow6"(w300) -> ()
                }
                frame 7 {
                  n336 = global write "GlobalReg.vi" "DMAsOverflow7"(w301) -> ()
                }
                frame 8 {
                  n337 = global write "GlobalReg.vi" "DMAsOverflow8"(w302) -> ()
                }
                frame 9 {
                  n338 = global write "GlobalReg.vi" "DMAsOverflow9"(w303) -> ()
                }
                frame 10 {
                  n339 = global write "GlobalReg.vi" "DMAsOverflow10"(w304) -> ()
                }
                frame 11 {
                  n340 = global write "GlobalReg.vi" "DMAsOverflow11"(w305) -> ()
                }
                frame 12 {
                  n341 = global write "GlobalReg.vi" "DMAsOverflow12"(w306) -> ()
                }
                frame 13 {
                  n342 = global write "GlobalReg.vi" "DMAsOverflow13"(w307) -> ()
                }
                frame 14 {
                  n343 = global write "GlobalReg.vi" "DMAsOverflow14"(w308) -> ()
                }
                frame 15 {
                  n344 = global write "GlobalReg.vi" "DMAsOverflow15"(w309) -> ()
                }
              }
              n345 = case shown="0, Default" w237 {
                tunnel: w226 -> [w278 w279 w280 w281 w282 w283 w284 w285 w286 w287 w288 w289 w290 w291 w292 w293]
                frame 0, Default {
                  n346 = global write "GlobalReg.vi" "DMAsOverflow0"(w278) -> ()
                }
                frame 1 {
                  n347 = global write "GlobalReg.vi" "DMAsOverflow1"(w279) -> ()
                }
                frame 2 {
                  n348 = global write "GlobalReg.vi" "DMAsOverflow2"(w280) -> ()
                }
                frame 3 {
                  n349 = global write "GlobalReg.vi" "DMAsOverflow3"(w281) -> ()
                }
                frame 4 {
                  n350 = global write "GlobalReg.vi" "DMAsOverflow4"(w282) -> ()
                }
                frame 5 {
                  n351 = global write "GlobalReg.vi" "DMAsOverflow5"(w283) -> ()
                }
                frame 6 {
                  n352 = global write "GlobalReg.vi" "DMAsOverflow6"(w284) -> ()
                }
                frame 7 {
                  n353 = global write "GlobalReg.vi" "DMAsOverflow7"(w285) -> ()
                }
                frame 8 {
                  n354 = global write "GlobalReg.vi" "DMAsOverflow8"(w286) -> ()
                }
                frame 9 {
                  n355 = global write "GlobalReg.vi" "DMAsOverflow9"(w287) -> ()
                }
                frame 10 {
                  n356 = global write "GlobalReg.vi" "DMAsOverflow10"(w288) -> ()
                }
                frame 11 {
                  n357 = global write "GlobalReg.vi" "DMAsOverflow11"(w289) -> ()
                }
                frame 12 {
                  n358 = global write "GlobalReg.vi" "DMAsOverflow12"(w290) -> ()
                }
                frame 13 {
                  n359 = global write "GlobalReg.vi" "DMAsOverflow13"(w291) -> ()
                }
                frame 14 {
                  n360 = global write "GlobalReg.vi" "DMAsOverflow14"(w292) -> ()
                }
                frame 15 {
                  n361 = global write "GlobalReg.vi" "DMAsOverflow15"(w293) -> ()
                }
              }
              n362 = xnode ("FIFO Write")("Element"=w244, "Timeout"=0, "FIFO In"=w235) -> ("Timed Out?"=w218:bool)  [unwired: 1 out]
              n363 = xnode ("FIFO Write")("Element"=w245, "Timeout"=0, "FIFO In"=w236) -> ("Timed Out?"=w213:bool)  [unwired: 1 out]
              n364 = feedback #9(FALSE) -> (w220:bool)
              n365 = Or(x=w220, y=w218) -> (x .or. y?=w221:bool)
              n366 = feedback-in #9(w221) -> ()
              n367 = feedback #10(FALSE) -> (w215:bool)
              n368 = Or(x=w215, y=w213) -> (x .or. y?=w216:bool)
              n369 = feedback-in #10(w216) -> ()
              n370 = case shown="0, Default" w233 {
                tunnel: w221 -> [w262 w263 w264 w265 w266 w267 w268 w269 w270 w271 w272 w273 w274 w275 w276 w277]
                frame 0, Default {
                  n371 = global write "GlobalReg.vi" "DMAsOverflow0"(w262) -> ()
                }
                frame 1 {
                  n372 = global write "GlobalReg.vi" "DMAsOverflow1"(w263) -> ()
                }
                frame 2 {
                  n373 = global write "GlobalReg.vi" "DMAsOverflow2"(w264) -> ()
                }
                frame 3 {
                  n374 = global write "GlobalReg.vi" "DMAsOverflow3"(w265) -> ()
                }
                frame 4 {
                  n375 = global write "GlobalReg.vi" "DMAsOverflow4"(w266) -> ()
                }
                frame 5 {
                  n376 = global write "GlobalReg.vi" "DMAsOverflow5"(w267) -> ()
                }
                frame 6 {
                  n377 = global write "GlobalReg.vi" "DMAsOverflow6"(w268) -> ()
                }
                frame 7 {
                  n378 = global write "GlobalReg.vi" "DMAsOverflow7"(w269) -> ()
                }
                frame 8 {
                  n379 = global write "GlobalReg.vi" "DMAsOverflow8"(w270) -> ()
                }
                frame 9 {
                  n380 = global write "GlobalReg.vi" "DMAsOverflow9"(w271) -> ()
                }
                frame 10 {
                  n381 = global write "GlobalReg.vi" "DMAsOverflow10"(w272) -> ()
                }
                frame 11 {
                  n382 = global write "GlobalReg.vi" "DMAsOverflow11"(w273) -> ()
                }
                frame 12 {
                  n383 = global write "GlobalReg.vi" "DMAsOverflow12"(w274) -> ()
                }
                frame 13 {
                  n384 = global write "GlobalReg.vi" "DMAsOverflow13"(w275) -> ()
                }
                frame 14 {
                  n385 = global write "GlobalReg.vi" "DMAsOverflow14"(w276) -> ()
                }
                frame 15 {
                  n386 = global write "GlobalReg.vi" "DMAsOverflow15"(w277) -> ()
                }
              }
              n387 = case shown="0, Default" w234 {
                tunnel: w216 -> [w246 w247 w248 w249 w250 w251 w252 w253 w254 w255 w256 w257 w258 w259 w260 w261]
                frame 0, Default {
                  n388 = global write "GlobalReg.vi" "DMAsOverflow0"(w246) -> ()
                }
                frame 1 {
                  n389 = global write "GlobalReg.vi" "DMAsOverflow1"(w247) -> ()
                }
                frame 2 {
                  n390 = global write "GlobalReg.vi" "DMAsOverflow2"(w248) -> ()
                }
                frame 3 {
                  n391 = global write "GlobalReg.vi" "DMAsOverflow3"(w249) -> ()
                }
                frame 4 {
                  n392 = global write "GlobalReg.vi" "DMAsOverflow4"(w250) -> ()
                }
                frame 5 {
                  n393 = global write "GlobalReg.vi" "DMAsOverflow5"(w251) -> ()
                }
                frame 6 {
                  n394 = global write "GlobalReg.vi" "DMAsOverflow6"(w252) -> ()
                }
                frame 7 {
                  n395 = global write "GlobalReg.vi" "DMAsOverflow7"(w253) -> ()
                }
                frame 8 {
                  n396 = global write "GlobalReg.vi" "DMAsOverflow8"(w254) -> ()
                }
                frame 9 {
                  n397 = global write "GlobalReg.vi" "DMAsOverflow9"(w255) -> ()
                }
                frame 10 {
                  n398 = global write "GlobalReg.vi" "DMAsOverflow10"(w256) -> ()
                }
                frame 11 {
                  n399 = global write "GlobalReg.vi" "DMAsOverflow11"(w257) -> ()
                }
                frame 12 {
                  n400 = global write "GlobalReg.vi" "DMAsOverflow12"(w258) -> ()
                }
                frame 13 {
                  n401 = global write "GlobalReg.vi" "DMAsOverflow13"(w259) -> ()
                }
                frame 14 {
                  n402 = global write "GlobalReg.vi" "DMAsOverflow14"(w260) -> ()
                }
                frame 15 {
                  n403 = global write "GlobalReg.vi" "DMAsOverflow15"(w261) -> ()
                }
              }
            }
          }
          n404 = case shown="True" w50 {
            tunnel: w64 -> [_ w324]
            frame False {
            }
            frame True {
              n405 = xnode ("FIFO Method Node")("Element"=w324, "Timeout"=0, "FIFO In"="IntermediateFIFO") -> ("Timed Out?"=w325:bool)  [unwired: 1 out]
              n406 = feedback #11(FALSE) -> (w327:bool)
              n407 = Or(x=w325, y=w327) -> (x .or. y?=w326:bool)
              n408 = feedback-in #11(w326) -> ()
              n409 = case shown="0, Default" "DMA number" {
                tunnel: w326 -> [w330 w331 w332 w333 w334 w335 w336 w337 w338 w339 w340 w341 w342 w343 w344 w345]
                frame 0, Default {
                  n410 = global write "GlobalReg.vi" "DMAsOverflow0"(w330) -> ()
                }
                frame 1 {
                  n411 = global write "GlobalReg.vi" "DMAsOverflow1"(w331) -> ()
                }
                frame 2 {
                  n412 = global write "GlobalReg.vi" "DMAsOverflow2"(w332) -> ()
                }
                frame 3 {
                  n413 = global write "GlobalReg.vi" "DMAsOverflow3"(w333) -> ()
                }
                frame 4 {
                  n414 = global write "GlobalReg.vi" "DMAsOverflow4"(w334) -> ()
                }
                frame 5 {
                  n415 = global write "GlobalReg.vi" "DMAsOverflow5"(w335) -> ()
                }
                frame 6 {
                  n416 = global write "GlobalReg.vi" "DMAsOverflow6"(w336) -> ()
                }
                frame 7 {
                  n417 = global write "GlobalReg.vi" "DMAsOverflow7"(w337) -> ()
                }
                frame 8 {
                  n418 = global write "GlobalReg.vi" "DMAsOverflow8"(w338) -> ()
                }
                frame 9 {
                  n419 = global write "GlobalReg.vi" "DMAsOverflow9"(w339) -> ()
                }
                frame 10 {
                  n420 = global write "GlobalReg.vi" "DMAsOverflow10"(w340) -> ()
                }
                frame 11 {
                  n421 = global write "GlobalReg.vi" "DMAsOverflow11"(w341) -> ()
                }
                frame 12 {
                  n422 = global write "GlobalReg.vi" "DMAsOverflow12"(w342) -> ()
                }
                frame 13 {
                  n423 = global write "GlobalReg.vi" "DMAsOverflow13"(w343) -> ()
                }
                frame 14 {
                  n424 = global write "GlobalReg.vi" "DMAsOverflow14"(w344) -> ()
                }
                frame 15 {
                  n425 = global write "GlobalReg.vi" "DMAsOverflow15"(w345) -> ()
                }
              }
            }
          }
        }
        frame 1, Default {
        }
      }
      n426 = Decrement(x=w19) -> (x-1=w20:u16)
      n427 = Increment(x=w16) -> (x+1=w22:u16)
      n428 = Less Or Equal?(x=w20, y=w16) -> (x <= y?=w23:bool)
      n429 = Select(t=u16 0, s=w23, f=w22) -> (s? t:f=w17:u16)
      n430 = xnode ("Register Write")("Data"=w17, "Register In"=w18) -> ()  [unwired: 1 out]
    }
  }
